vi "Stop Core.vi"(10 "final error code":i32, 11 "Coffee Shop in":refnum<class "Coffee Shop.lvclass">) -> (3 "Coffee Shop out":refnum<class "Coffee Shop.lvclass">)   [LabVIEW 2023, in "Coffee Shop.lvlib" / "Coffee Shop.lvclass"]
doc: "(<B>Filename</B>: Actor Framework.lvlib:Actor.lvclass:Stop Core.vi)\n\nDefines what the actor does before it stops. Use the <B>final error code</B> input to determine whether the actor shut down in response to an error.\n\nBy default, this method does nothing. A descendant class may override it to define behavior, such as shutting down any processes the actor initiated in its override of the Actor Core method."
uses:
  Coffee Shop.lvclass
  Coffee Shop.lvclass/Coffee Shop.ctl
  <vilib>/ActorFramework/Actor/Actor.lvclass
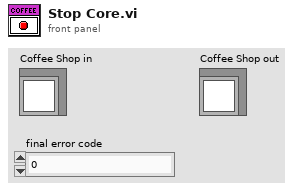
[diagram p1: front panel]
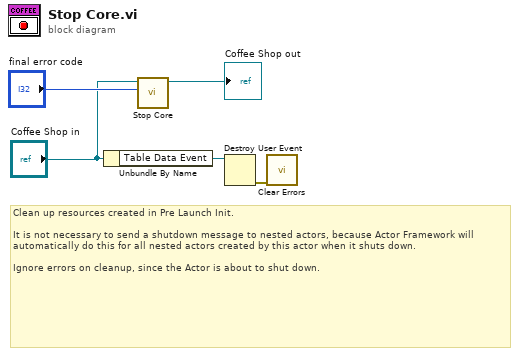
[diagram p0: block diagram]
diagram:
  # "Clean up resources created in Pre Launch Init.\n\nIt is not necessary to send a shutdown message to nested actors, because Actor Framework will automatically do this for all nested actors created by this actor when it shuts down.\n\nIgnore errors on cleanup, since the Actor is about to shut down."
  n1 = Unbundle By Name("Coffee Shop in") -> ("Table Data Event"=w3:refnum<user-event>)
  n2 = call-parent "Stop Core.vi"("final error code"="final error code", "Actor in"="Coffee Shop in") -> ("Actor out"=→"Coffee Shop out":refnum<class "Coffee Shop.lvclass">)  [unwired: 9 in]
  n3 = Destroy User Event(user event=w3) -> (error out=w1:errorcluster)  [unwired: 1 in]
  n4 = call <vilib>:"Clear Errors.vi"("error in (no error)"=w1) -> ()  [unwired: 5 in, 2 out]
